vi "Microsync create packet.vi"(1 "interval_us":u32, 2 "Command":string, 3 "N":u32, 4 "timestamp_us":u32, 5 "arg2":u32, 6 "arg1":u32) -> (0 "data packet":string)   [LabVIEW 2023]
panel:
  out "length":i32
  out "arguments":string
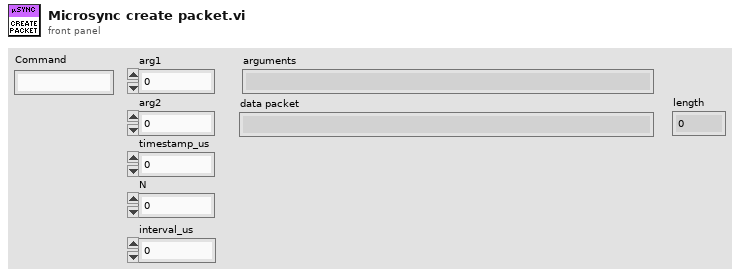
[diagram p1: front panel]
types:
  T1 = enum16{"big-endian, network order", "native, host order", "little-endian"}
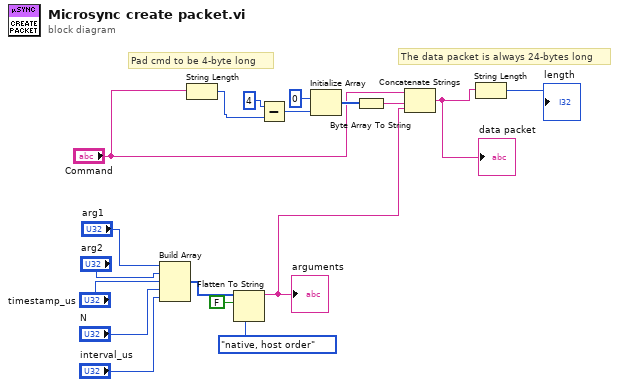
[diagram p0: block diagram]
diagram:
  # "Pad cmd to be 4-byte long"
  # "The data packet is always 24-bytes long"
  n1 = Build Array("arg1", "arg2", "timestamp_us", "N", "interval_us") -> (w2:u32[])
  n2 = String Length(string="Command") -> (length=w9:i32)
  n3 = Flatten To String(anything=w2, prepend array or string size? (T)=FALSE, byte order (0:big-endian, network order)=T1."native, host order") -> (data string=w3:string)  [unwired: 1 in, 2 out]
  "arguments" <- w3
  n4 = Subtract(x=4, y=w9) -> (x-y=w8:i32)
  n5 = Initialize Array(u8 0 ("element"), w8) -> (w10:u8[])
  n6 = Byte Array To String(unsigned byte array=w10) -> (string=w11:string)
  n7 = Concatenate Strings("Command", w11, w3) -> (w1:string)
  "data packet" <- w1
  n8 = String Length(string=w1) -> (length=→"length":i32)
